vi "ConstructorString.vi"(6 "error in":errorcluster, 9 "Diagram in":refnum<class "Diagram.lvclass">) -> (0 "error out":errorcluster, 3 "Diagram out":refnum<class "Diagram.lvclass">, 4 "constructor":string)   [LabVIEW 2014, in "Raspberry Pi Compatible Compiler for LabVIEW.lvlib" / "Diagram.lvclass"]
uses:
  Diagram.lvclass
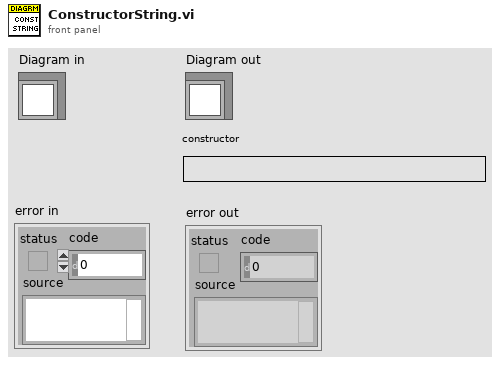
[diagram p1: front panel]
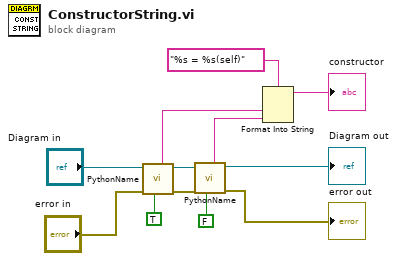
[diagram p0: block diagram]
diagram:
  n1 = call-dynamic "PythonName.vi"("add self"=TRUE, "error in"="error in", "Diagram in"="Diagram in") -> ("error out"=w10:errorcluster, "Diagram out"=w9:refnum<class "Diagram.lvclass">, "name"=w4:string)  [unwired: 5 in, 1 out]
  n2 = call-dynamic "PythonName.vi"("add self"=FALSE, "error in"=w10, "Diagram in"=w9) -> ("error out"=→"error out":errorcluster, "Diagram out"=→"Diagram out":refnum<class "Diagram.lvclass">, "name"=w5:string)  [unwired: 5 in, 1 out]
  n3 = Format Into String(format string="%s = %s(self)", w4, w5) -> (resulting string=→"constructor":string)  [unwired: 2 in, 1 out]
